vi "PH_Beamline_Common.set MM1 Bend.vi"(2 "CtlRef":refnum<vi>, 3 "State":T1 items=["unknown", "Position I", "Position II", "Position III", "Position IV", "moving"], 4 "no link":bool, 5 "error in (no error)":errorcluster) -> (19 "error out":errorcluster)   [LabVIEW 2014, in "PH_Beamline_Common.lvlib"]
uses:
  PH_Beamline_Common.lvlib
  PH_Motion/PH_4_Pos_Selector/PH_4_Pos_Selector.Position Selector.ctl
  PH_Common/PH_Common.lvlib
  PH_Motion/PH_4_Pos_Selector/PH_4_Pos_Selector.lvlib
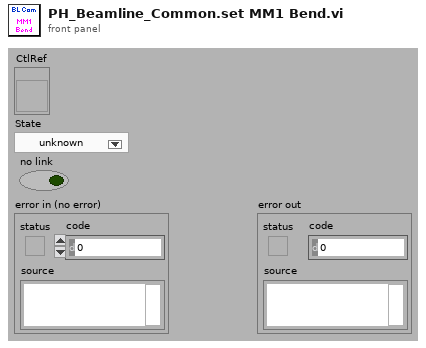
[diagram p1: front panel]
types:
  T1 = typedef "PH_4_Pos_Selector.lvlib/PH_4_Pos_Selector.Position Selector.ctl" = u16
  T2 = cluster{"horizontal":enum16{"left", "center", "right"}, "vertical":enum16{"top", "center", "bottom"}}
  T3 = cluster{"left":i16, "top":i16, "right":i16, "bottom":i16}
  T4 = cluster{"Width":u16, "Style":enum32{"Solid", "Dash", "Dot", "DashDot", "DashDotDot"}}
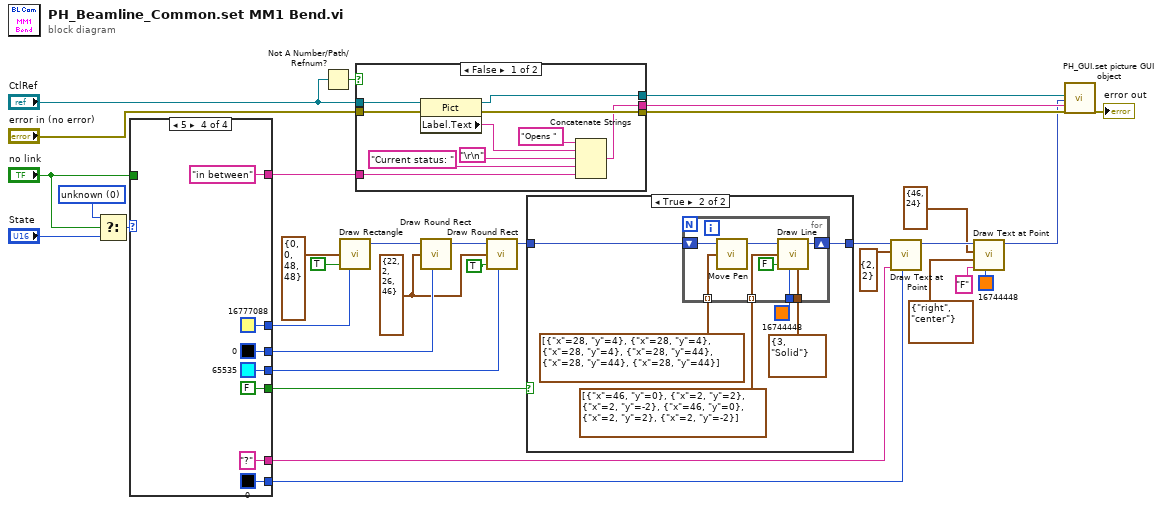
[diagram p0: block diagram]
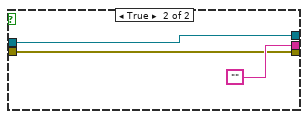
[diagram p3: hidden frame]
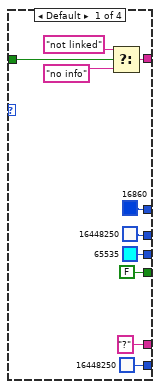
[diagram p4: hidden frame]
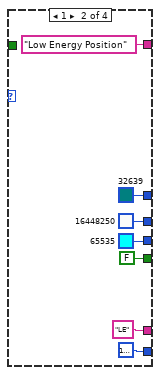
[diagram p5: hidden frame]
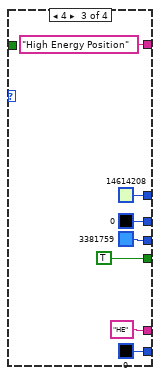
[diagram p6: hidden frame]
diagram:
  w11 = T3 {"left"=22, "top"=2, "right"=26, "bottom"=46} ("rect")
  w13 = T1 0 items=["unknown", "Position I", "Position II", "Position III", "Position IV", "moving"] ("State")
  n1 = Select(t=w13, s="no link", f="State") -> (s? t:f=w24:T1)
  n2 = case shown="5" w24 {
    tunnel: [u32 16860 u32 32639 u32 14614208 u32 16777088] -> w27
    tunnel: "no link" -> [w39 _ _ _]
    tunnel: [w40 "Low Energy Position" "High Energy Position" "in between"] -> w23
    tunnel: [u32 16448250 u32 16448250 u32 0 u32 0] -> w17
    tunnel: ["?" "LE" "HE" "?"] -> w18
    tunnel: [u32 16448250 u32 16777226 u32 0 u32 0] -> w16
    tunnel: [FALSE FALSE TRUE FALSE] -> w8
    tunnel: [u32 65535 u32 65535 u32 3381759 u32 65535] -> w7
    frame Default {
      n3 = Select(t="not linked", s=w39, f="no info") -> (s? t:f=w40:string)
    }
    frame 1 {
    }
    frame 4 {
    }
    frame 5 {
    }
  }
  n4 = Not A Number/Path/Refnum?(number/path/refnum="CtlRef") -> (NaN/Path/Refnum?=w14:bool)
  n5 = call <vilib>:"Draw Rectangle.vi"("rect"=T3 {"left"=0, "top"=0, "right"=48, "bottom"=48}, "fill?(F)"=TRUE, "color(black)"=w27) -> ("new picture"=w20:picture)  [unwired: 6 in]
  n6 = case shown="False" w14 {
    tunnel: "CtlRef" -> [w70 w77]
    tunnel: "error in (no error)" -> [w69 w75]
    tunnel: [w68 w75] -> w25
    tunnel: w23 -> [w67 _]
    tunnel: [w66 ""] -> w22
    tunnel: [w65 w77] -> w15
    frame False {
      n7 = property class="Pict"(reference=w70, error in=w69) -> (reference out=w65:refnum<vi>, error out=w68:errorcluster, "Label.Text"=w73:string)
      n8 = Concatenate Strings("Opens " ("string"), w73, "\r\n", "Current status: " ("string"), w67) -> (w66:string)
    }
    frame True {
    }
  }
  n9 = call <vilib>:"Draw Round Rect.vi"("picture"=w20, "rect"=w11, "color(black)"=w17) -> ("new picture"=w19:picture)  [unwired: 6 in]
  n10 = call <vilib>:"Draw Round Rect.vi"("picture"=w19, "rect"=w11, "fill?(F)"=TRUE, "color(black)"=w7) -> ("new picture"=w10:picture)  [unwired: 5 in]
  n11 = case shown="True" w8 {
    tunnel: w10 -> [w78 w84]
    tunnel: [w78 w83] -> w9
    frame False {
    }
    frame True {
      n12 = for {
        tunnel: u32 16744448 ("color(black)") -> [w91]
        tunnel: T4 {"Width"=3, "Style"=enum."Solid"} ("pen") -> [w90]
        tunnel: cluster{"x":i16, "y":i16}[] [{"x"=28, "y"=4}, {"x"=28, "y"=4}, {"x"=28, "y"=4}, {"x"=28, "y"=44}, {"x"=28, "y"=44}, {"x"=28, "y"=44}] -> [w86] mode=indexing
        shift-right: [w92] -> w83
        shift-left: w84 -> [w89]
        tunnel: cluster{"x":i16, "y":i16}[] [{"x"=46, "y"=0}, {"x"=2, "y"=2}, {"x"=2, "y"=-2}, {"x"=46, "y"=0}, {"x"=2, "y"=2}, {"x"=2, "y"=-2}] -> [w85] mode=indexing
        n13 = call <vilib>:"Move Pen.vi"("new position"=w86, "picture"=w89) -> ("new picture"=w88:picture)  [unwired: 3 in]
        n14 = call <vilib>:"Draw Line.vi"("picture"=w88, "end point"=w85, "absolute coordinates?(T)"=FALSE, "color(black)"=w91, "pen"=w90) -> ("new picture"=w92:picture)  [unwired: 4 in]
      }
    }
  }
  n15 = call <vilib>:"Draw Text at Point.vi"("text color(black)"=w16, "text"=w18, "origin"=cluster{"x":i16, "y":i16} {"x"=2, "y"=2}, "picture"=w9) -> ("new picture"=w6:picture)  [unwired: 6 in, 1 out]
  n16 = call <vilib>:"Draw Text at Point.vi"("text color(black)"=u32 16744448, "text"="F", "alignment(left, top)"=T2 {"horizontal"=enum."right", "vertical"=enum."center"}, "origin"=cluster{"x":i16, "y":i16} {"x"=46, "y"=24}, "picture"=w6) -> ("new picture"=w5:picture)  [unwired: 5 in, 1 out]
  n17 = call "PH_GUI.set picture GUI object.vi"("CtlRef"=w15, "Picture"=w5, "Tip Strip (\"\")"=w22, "error in (no error)"=w25) -> ("error out"=→"error out":errorcluster)  [unwired: 15 in]
